vi "多列表初始化.vi"(7 "配置文件路径":path=path "C:/Users/Azmat/Desktop/Labview/发送协议.txt", 9 "多列列表框":refnum<vi>) -> (3 "发送配置":T1(array[cluster]))   [LabVIEW 2016]
uses:
  <vilib>/Utility/miscctls.llb/LVRowAndColumnTypeDef.ctl
panel:
  out "floor(x/y)":i32
  out "大小":i32
  out "数组":string[][](array[string])
  in  "end pattern string":string="#end"
  in  "start pattern string":string="#start"
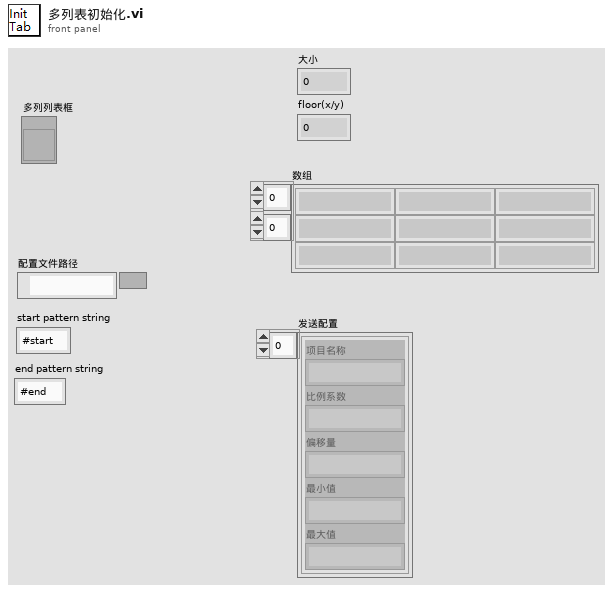
[diagram p1: front panel]
types:
  T1 = cluster{"项目名称":string, "比例系数":string, "偏移量":string, "最小值":string, "最大值":string}[]
  T2 = typedef "LVRowAndColumnTypeDef.ctl" = cluster{"Row":i32, "Column":i32}
  T3 = cluster{"项目名称":string, "比例系数":string, "偏移量":string, "最小值":string, "最大值":string}
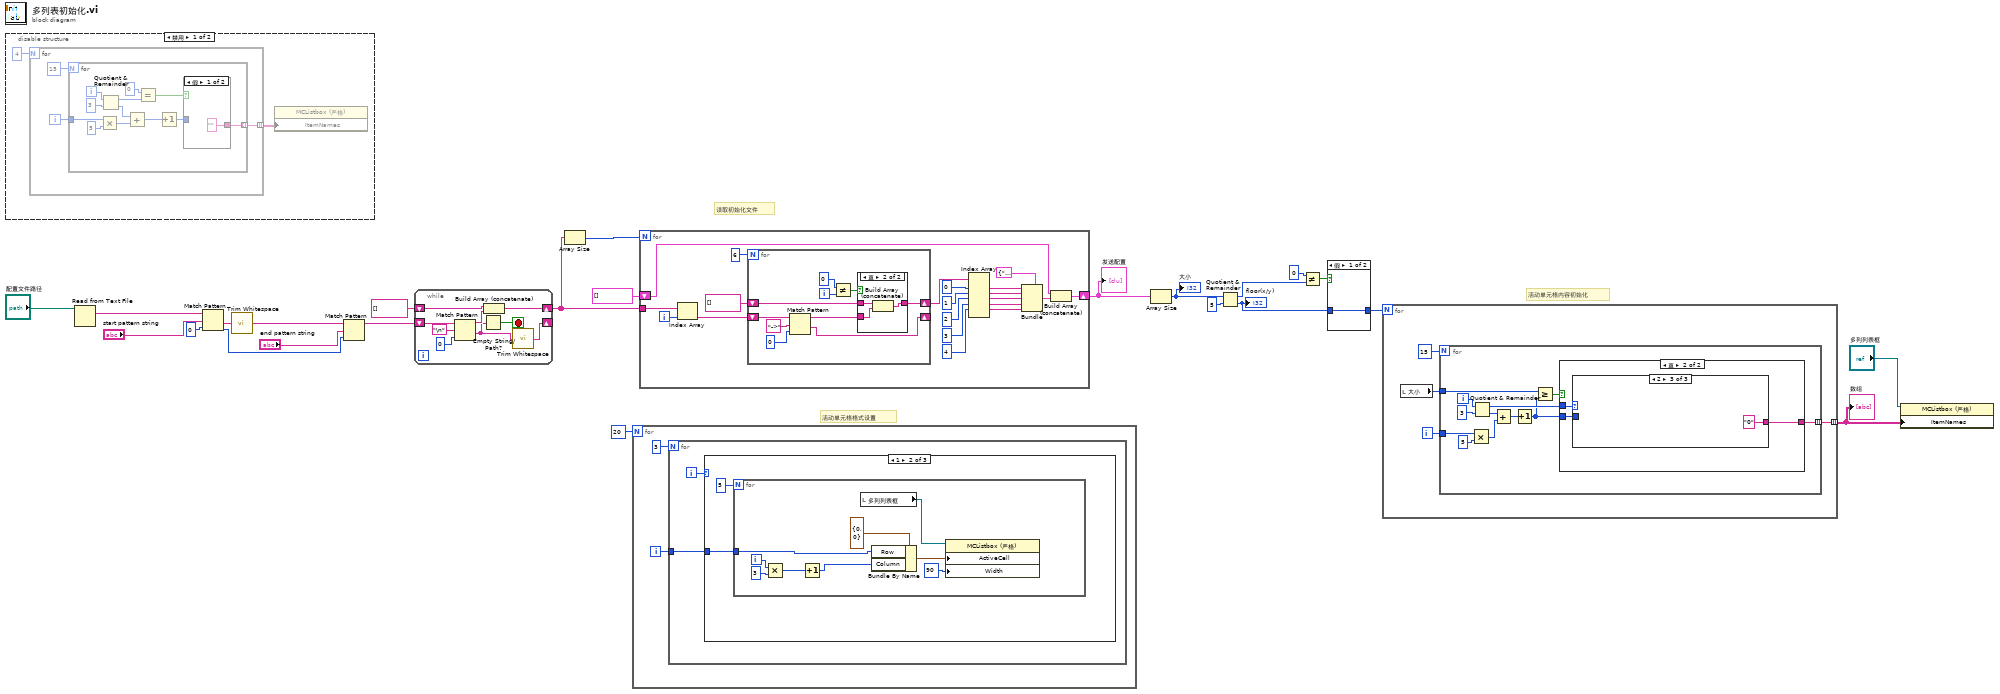
[diagram p0: block diagram]
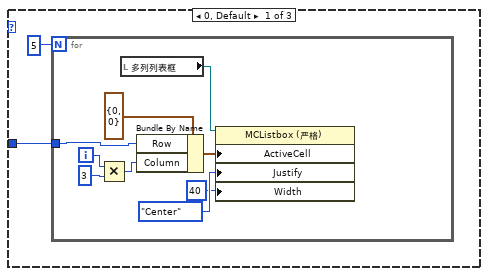
[diagram p2: hidden frame]
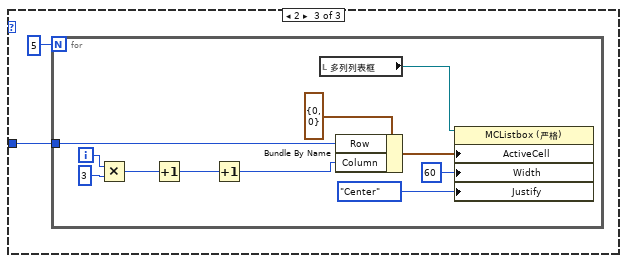
[diagram p3: hidden frame]
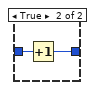
[diagram p4: hidden frame]
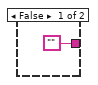
[diagram p5: hidden frame]
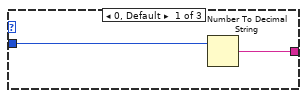
[diagram p6: hidden frame]
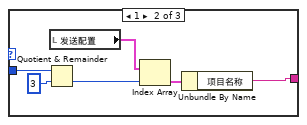
[diagram p7: hidden frame]
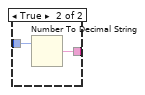
[diagram p9: hidden frame]
diagram:
  # "读取初始化文件"
  # "活动单元格内容初始化"
  # "活动单元格格式设置"
  n1 = disable-structure shown="禁用" {
    frame Disabled {
      n2 = for {
        N: 4 -> [_]
        tunnel: [w30] -> w27 mode=indexing
        i -> [w28]
        n3 = for {
          N: 15 -> [_]
          tunnel: [w42] -> w30 mode=indexing
          tunnel: w28 -> [w33]
          i -> [w36]
          n4 = Multiply(x=w33, y=5) -> (x*y=w31:i32)
          n5 = Quotient & Remainder(x=w36, y=3) -> (x-y*floor(x/y)=w40:i32, floor(x/y)=w34:i32)
          n6 = Add(x=w34, y=w31) -> (x+y=w35:i32)
          n7 = Equal?(x=0, y=w40) -> (x = y?=w38:bool)
          n8 = Increment(x=w35) -> (x+1=w37:i32)
          n9 = case shown="假" w38 {
            tunnel: ["" w45] -> w42
            tunnel: w37 -> [_ w44]
            frame False {
            }
            frame True {
              n10 = Number To Decimal String(number=w44) -> (decimal integer string=w45:string)  [unwired: 1 in]
            }
          }
        }
      }
      n11 = property on="属性节点" class="MCListbox (严格)"("ItemNames"=w27) -> (reference=w25:refnum<vi>)  [unwired: 1 in, 2 out]
    }
    frame Enabled {
    }
  }
  n12 = Read from Text File(file (use dialog)="配置文件路径") -> (text=w23:string)  [unwired: 3 in, 3 out]
  n13 = Match Pattern(string=w23, regular expression="start pattern string", offset (0)=0) -> (after substring=w17:string, offset past match=w20:i32)  [unwired: 2 out]
  n14 = call <vilib>:"Trim Whitespace.vi"("string"=w17) -> ("trimmed string"=w18:string)  [unwired: 1 in]
  n15 = Match Pattern(string=w18, regular expression="end pattern string", offset (0)=w20) -> (before substring=w15:string)  [unwired: 3 out]
  n16 = while {
    shift-right: [w51] -> w13
    shift-left: string[] [] ("appended array") -> [w52]
    shift-right: [w48] -> _
    shift-left: w15 -> [w50]
    stop <- w54 stop-if-true
    n17 = Match Pattern(string=w50, regular expression="\n", offset (0)=0) -> (before substring=w53:string, after substring=w49:string)  [unwired: 2 out]
    n18 = Empty String/Path?(string/path=w49) -> (empty?=w54:bool)
    n19 = Build Array (concatenate)(w52, w53) -> (w51:string[])
    n20 = call <vilib>:"Trim Whitespace.vi"("string"=w49) -> ("trimmed string"=w48:string)  [unwired: 1 in]
  }
  n21 = Array Size(array=w13) -> (size(s)=w14:i32)
  n22 = for {
    N: 20 -> [_]
    i -> [w55]
    n23 = for {
      N: 3 -> [_]
      tunnel: w55 -> [w57]
      i -> [w58]
      n24 = case shown="1" w58 {
        tunnel: w57 -> [w59 w70 w81]
        frame 0, Default {
          n25 = for {
            N: 5 -> [_]
            tunnel: w59 -> [w62]
            i -> [w67]
            n26 = Multiply(x=w67, y=3) -> (x*y=w65:i32)
            n27 = local read "多列列表框"() -> (w64:refnum<vi>)
            n28 = Bundle By Name(cluster=T2 {"Row"=0, "Column"=0} ("活动单元格:活动单元格"), "Row"=w62, "Column"=w65) -> (w68:T2)
            n29 = property class="MCListbox (严格)"(reference=w64, "ActiveCell"=w68, "Justify"=enum16{"Left", "Center", "Right"}."Center" ("活动单元格:单元格对齐"), "Width"=u32 40 ("活动单元格:单元格大小:宽度")) -> ()  [unwired: 1 in, 2 out]
          }
        }
        frame 1 {
          n30 = for {
            N: 5 -> [_]
            tunnel: w70 -> [w72]
            i -> [w76]
            n31 = Multiply(x=w76, y=3) -> (x*y=w74:i32)
            n32 = Increment(x=w74) -> (x+1=w73:i32)
            n33 = local read "多列列表框"() -> (w79:refnum<vi>)
            n34 = Bundle By Name(cluster=T2 {"Row"=0, "Column"=0} ("活动单元格:活动单元格"), "Row"=w72, "Column"=w73) -> (w77:T2)
            n35 = property class="MCListbox (严格)"(reference=w79, "ActiveCell"=w77, "Width"=u32 90 ("活动单元格:单元格大小:宽度")) -> ()  [unwired: 1 in, 2 out]
          }
        }
        frame 2 {
          n36 = for {
            N: 5 -> [_]
            tunnel: w81 -> [w83]
            i -> [w90]
            n37 = Multiply(x=w90, y=3) -> (x*y=w88:i32)
            n38 = Increment(x=w88) -> (x+1=w86:i32)
            n39 = Increment(x=w86) -> (x+1=w85:i32)
            n40 = local read "多列列表框"() -> (w87:refnum<vi>)
            n41 = Bundle By Name(cluster=T2 {"Row"=0, "Column"=0} ("活动单元格:活动单元格"), "Row"=w83, "Column"=w85) -> (w91:T2)
            n42 = property class="MCListbox (严格)"(reference=w87, "ActiveCell"=w91, "Width"=u32 60 ("活动单元格:单元格大小:宽度"), "Justify"=enum16{"Left", "Center", "Right"}."Center" ("活动单元格:单元格对齐")) -> ()  [unwired: 1 in, 2 out]
          }
        }
      }
    }
  }
  n43 = for {
    N: w14 -> [_]
    tunnel: w13 -> [w113]
    shift-right: [w97] -> w11
    shift-left: T1 [] -> [w96]
    i -> [w98]
    n44 = Index Array(array=w113, index=w98) -> (element=w111:string)
    n45 = for {
      N: 6 -> [_]
      shift-right: [w120] -> _
      shift-left: w111 -> [w121]
      shift-right: [w117] -> w109
      shift-left: string[] [] -> [w118]
      i -> [w116]
      n46 = Match Pattern(string=w121, regular expression="->", offset (0)=0) -> (before substring=w119:string, after substring=w120:string)  [unwired: 2 out]
      n47 = Not Equal?(x=0, y=w116) -> (x != y?=w114:bool)
      n48 = case shown="真" w114 {
        tunnel: w119 -> [_ w127]
        tunnel: w118 -> [w124 w126]
        tunnel: [w124 w125] -> w117
        frame False {
        }
        frame True {
          n49 = Build Array (concatenate)(w126, w127) -> (w125:string[])
        }
      }
    }
    n50 = Index Array(array=w109, index #1=0 ("index"), index #2=1 ("index"), index #3=2 ("index"), index #4=3 ("index"), index #5=4 ("index")) -> (element #1=w108:string, element #2=w102:string, element #3=w101:string, element #4=w100:string, element #5=w99:string)  [unwired: 1 in, 1 out]
    n51 = Bundle(cluster=T3 {"项目名称"="", "比例系数"="", "偏移量"="", "最小值"="", "最大值"=""} ("Cluster"), "项目名称"=w108, "比例系数"=w102, "偏移量"=w101, "最小值"=w100, "最大值"=w99) -> (w94:T3)
    n52 = Build Array (concatenate)(w96, w94) -> (w97:T1)
  }
  "发送配置" <- w11
  n53 = Array Size(array=w11) -> (size(s)=w9:i32)
  "大小" <- w9
  n54 = Quotient & Remainder(x=w9, y=5) -> (x-y*floor(x/y)=w6:i32, floor(x/y)=w4:i32)
  "floor(x/y)" <- w4
  n55 = Not Equal?(x=0, y=w6) -> (x != y?=w8:bool)
  n56 = case shown="假" w8 {
    tunnel: w4 -> [w128 w130]
    tunnel: [w128 w129] -> w5
    frame False {
    }
    frame True {
      n57 = Increment(x=w130) -> (x+1=w129:i32)
    }
  }
  n58 = for {
    N: w5 -> [_]
    tunnel: [w133] -> w2 mode=indexing
    i -> [w134]
    n59 = local read "大小"() -> (w131:i32)
    n60 = for {
      N: 15 -> [_]
      tunnel: [w146] -> w133 mode=indexing
      tunnel: w134 -> [w141]
      tunnel: w131 -> [w135]
      i -> [w144]
      n61 = Multiply(x=w141, y=5) -> (x*y=w139:i32)
      n62 = Quotient & Remainder(x=w144, y=3) -> (x-y*floor(x/y)=w138:i32, floor(x/y)=w142:i32)
      n63 = Add(x=w142, y=w139) -> (x+y=w143:i32)
      n64 = Increment(x=w143) -> (x+1=w136:i32)
      n65 = Greater Or Equal?(x=w135, y=w136) -> (x >= y?=w137:bool)
      n66 = case shown="真" w137 {
        tunnel: ["" w150] -> w146
        tunnel: w136 -> [_ w149]
        tunnel: w138 -> [_ w148]
        frame False {
        }
        frame True {
          n67 = case shown="2" w148 {
            tunnel: [w151 w153 "0"] -> w150
            tunnel: w149 -> [w152 w157 _]
            frame 0, Default {
              n68 = Number To Decimal String(number=w152) -> (decimal integer string=w151:string)  [unwired: 1 in]
            }
            frame 1 {
              n69 = Quotient & Remainder(x=w157, y=3) -> (floor(x/y)=w156:i32)  [unwired: 1 out]
              n70 = local read "发送配置"() -> (w158:T1)
              n71 = Index Array(array=w158, index=w156) -> (element=w154:T3)
              n72 = Unbundle By Name(w154) -> ("项目名称"=w153:string)
            }
            frame 2 {
            }
          }
        }
      }
    }
  }
  "数组" <- w2
  n73 = property class="MCListbox (严格)"(reference="多列列表框", "ItemNames"=w2) -> ()  [unwired: 1 in, 2 out]
